vi "niRFSysCalReader Fetch Cal Info.vi"(8 "error in":errorcluster, 11 "niRFSysCalReader Handle":T2) -> (0 "error out":errorcluster, 2 "Cal Info":T1, 3 "niRFSysCalReader Handle out":T2)   [LabVIEW 2016, in "niRFSysCalReader.lvlib"]
doc: "Returns general information about the system calibration."
uses:
  niRFSysCalReader.lvlib
  INCLUDES/niRFSysCalReader Handle.ctl
  INCLUDES/niRFSysCalReader CalPath Info.ctl
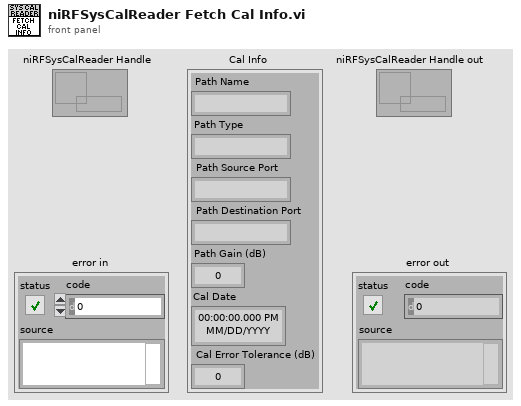
[diagram p1: front panel]
types:
  T1 = typedef "niRFSysCalReader.lvlib/niRFSysCalReader CalPath Info.ctl" = cluster{"Path Name":string, "Path Type":string, "Path Source Port":string, "Path Destination Port":string, "Path Gain (dB)":dbl, "Cal Date":timestamp, "Cal Error Tolerance (dB)":dbl}
  T2 = typedef "niRFSysCalReader.lvlib/niRFSysCalReader Handle.ctl" = refnum<data-value>
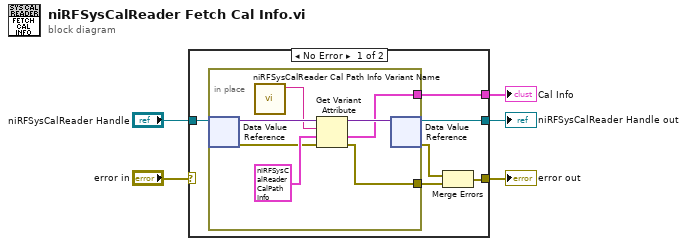
[diagram p0: block diagram]
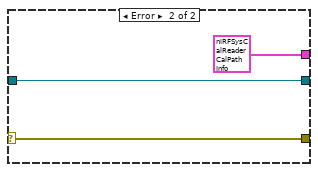
[diagram p2: hidden frame]
diagram:
  n1 = case shown="No Error" "error in" {
    selector: "error in" -> [_ w21]
    tunnel: [w11 w20] -> w5
    tunnel: "niRFSysCalReader Handle" -> [w10 w20]
    tunnel: [w9 w21] -> w2
    tunnel: [w6 T1 {"Path Name"="", "Path Type"="", "Path Source Port"="", "Path Destination Port"="", "Path Gain (dB)"=nan, "Cal Date"=timestamp(0 s since 1904-01-01), "Cal Error Tolerance (dB)"=nan} ("CalPath Info")] -> w1
    frame No Error {
      n2 = in-place {
        in-place-border: [w15] -> w7
        in-place-border: [w12] -> w6
        n3 = in-place-dvr #1(w10) -> (w18:variant, w13:errorcluster)
        n4 = call "niRFSysCalReader Cal Path Info Variant Name.vi"() -> ("Cal Path Info Name"=w17:string)  [unwired: 11 in]
        n5 = Get Variant Attribute(Variant=w18, name=w17, default value (empty Variant)=T1 {"Path Name"="", "Path Type"="", "Path Source Port"="", "Path Destination Port"="", "Path Gain (dB)"=0.0, "Cal Date"=timestamp(0 s since 1904-01-01), "Cal Error Tolerance (dB)"=0.0} ("CalPath Info"), error in=w13) -> (duplicate Variant=w16:variant, value=w12:T1, error out=w15:errorcluster)  [unwired: 1 out]
        n6 = in-place-dvr #1(w16) -> (w11:T2, w8:errorcluster)
      }
      n7 = Merge Errors(w8, w7) -> (w9:errorcluster)
    }
    frame Error {
    }
  }
  "niRFSysCalReader Handle out" <- w5
  "error out" <- w2
  "Cal Info" <- w1
